vi "add_alignment_center_ring.vi"(9 "Color":u32, 10 "center radius":dbl, 11 "Refnum in":T1) -> (3 "Refnum out":T1)   [LabVIEW 2011]
uses:
  <vilib>/vision/Image Controls.llb/IMAQ Image.ctl
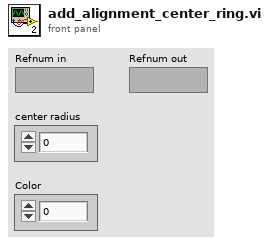
[diagram p1: front panel]
types:
  T1 = typedef "IMAQ Image.ctl" = refnum<image>
  T2 = cluster{"Numeric Control":dbl, "Numeric Control":dbl, "Numeric Control":dbl, "Numeric Control":dbl}
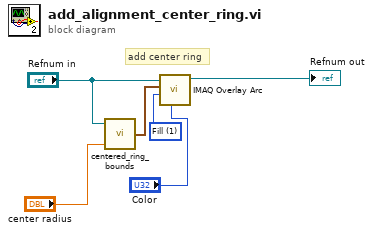
[diagram p0: block diagram]
diagram:
  w3 = u32 1 items=["Frame", "Fill"] ("Drawing Mode (Frame)")
  # "add center ring"
  n1 = call "centered_ring_bounds.vi"("radius R"="center radius", "Image"="Refnum in") -> ("Bounding Rectangle"=w1:T2)  [unwired: 3 in]
  n2 = call "IMAQ Overlay Arc"("Color"="Color", "Drawing Mode (Frame)"=w3, "Bounding Rectangle"=w1, "Image"="Refnum in") -> ("Image Out"=→"Refnum out":T1)  [unwired: 6 in, 1 out]
